vi "Wrapper.vi"(0 "measurement configuration":T1={"Channel(s)"="Lorem ipsum dolor sit", "Simulate?"=TRUE, "resource name Pin"=""}, 5 "resource name":refnum<k15>="Dev1" caption="Resource Name(s)", 11 "error in":errorcluster) -> (4 "measurement results":T2, 15 "error out":errorcluster)   [LabVIEW 2021, in "niScope EX Getting Started.lvlib"]
uses:
  niScope EX Getting Started.lvlib
  Measurement Results.ctl
  Measurement Configuration.ctl
  MeasurementCore/niScope EX Getting Started_dependencies.lvlib
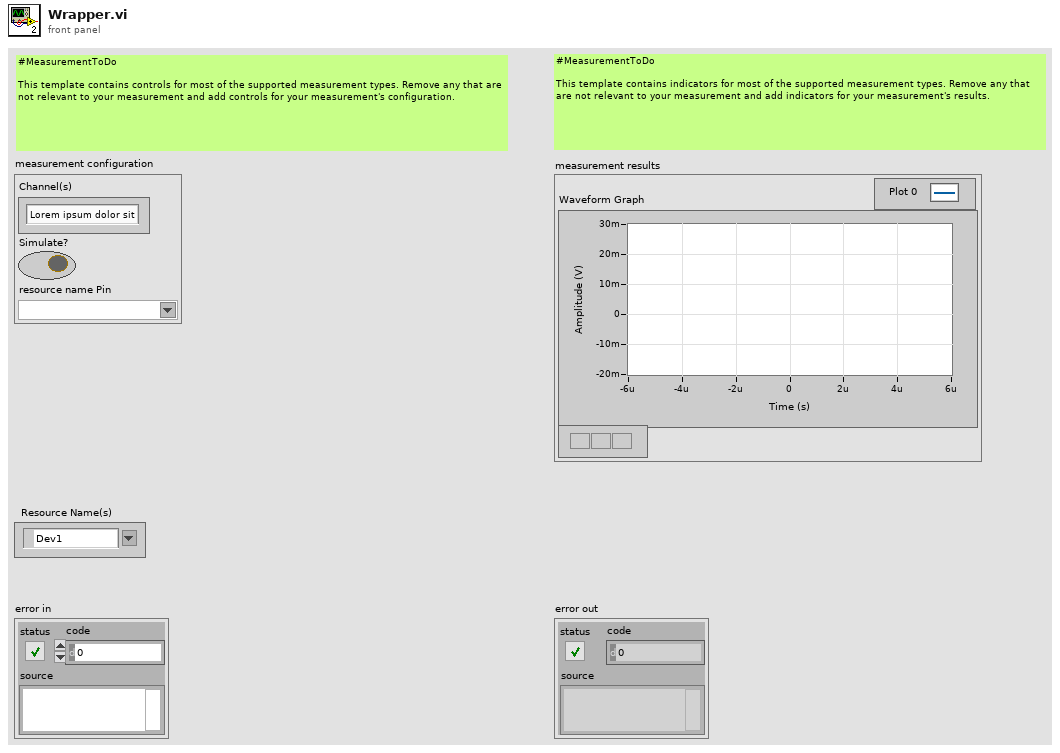
[diagram p1: front panel]
types:
  T1 = typedef "niScope EX Getting Started.lvlib/Measurement Configuration.ctl" = cluster{"Channel(s)":string, "Simulate?":bool, "resource name Pin":string}
  T2 = typedef "niScope EX Getting Started.lvlib/Measurement Results.ctl" = cluster{"Waveform Graph":cluster{"relativeInitialX":dbl, "xIncrement":dbl, "wfm":dbl[]}[]}
  T3 = cluster{"relativeInitialX":dbl, "xIncrement":dbl, "wfm":dbl[]}[]
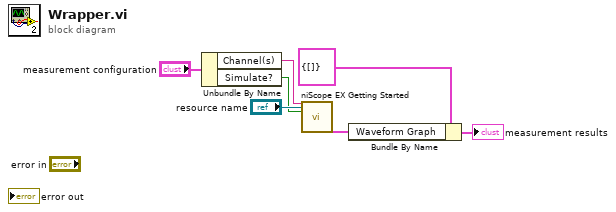
[diagram p0: block diagram]
diagram:
  n1 = Unbundle By Name("measurement configuration") -> ("Channel(s)"=w2:string, "Simulate?"=w1:bool)
  n2 = call "niScope EX Getting Started.vi"("Channel(s)"=w2, "resource name"="resource name", "Simulate?"=w1) -> ("Waveform Graph"=w5:T3)  [unwired: 24 in]
  n3 = Bundle By Name(cluster=T2 {"Waveform Graph"=[]} ("measurement results"), "Waveform Graph"=w5) -> (→"measurement results":T2)
